vi "Reset.vi"(8 "error in (no error)":errorcluster, 11 "Mod Admin in":refnum<class "ModuleAdminBase.lvclass">) -> (0 "error out":errorcluster, 3 "Mod Admin out":refnum<class "ModuleAdminBase.lvclass">)   [LabVIEW 2018, in "ModuleAdmin.lvlib" / "ModuleAdminBase.lvclass"]
uses:
  ModuleAdminBase.lvclass
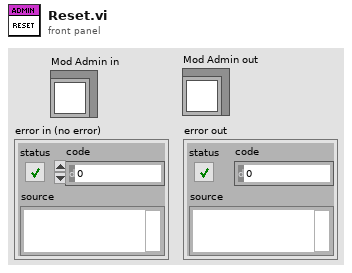
[diagram p1: front panel]
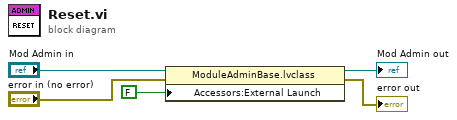
[diagram p0: block diagram]
diagram:
  n1 = property class="ModuleAdminBase.lvclass"(reference="Mod Admin in", error in="error in (no error)", "Accessors:External Launch"=FALSE) -> (reference out=→"Mod Admin out":refnum<class "ModuleAdminBase.lvclass">, error out=→"error out":errorcluster)
